vi "Delay in DDS.vi"() -> ()   [LabVIEW 2014]
uses:
  <vilib>/Platform/TimedLoop/XDataNode/timing_clust.ctl
  <vilib>/Platform/TimedLoop/XDataNode/nitl_modes.ctl
  <vilib>/Platform/TimedLoop/XDataNode/wakeup.ctl
  <vilib>/platform/TimedLoop/XDataNode/XDataNode.xnode
  <vilib>/Platform/TimedLoop/XDataNode/XDNodeRunTimeDep.lvlib
panel:
  out "x-y":u32
  out "millisecond timer value 2":u32
  out "millisecond timer value":u32
  out "Source vs PLC":cluster{"Value":dbl, "Value":dbl}(graph)
  out "PLC":dbl(graph)
  in  "PLC Scan Time":i64
  in  "DDS Update Rate":i64
  out "DDS":dbl(graph)
  out "Source":dbl(graph)
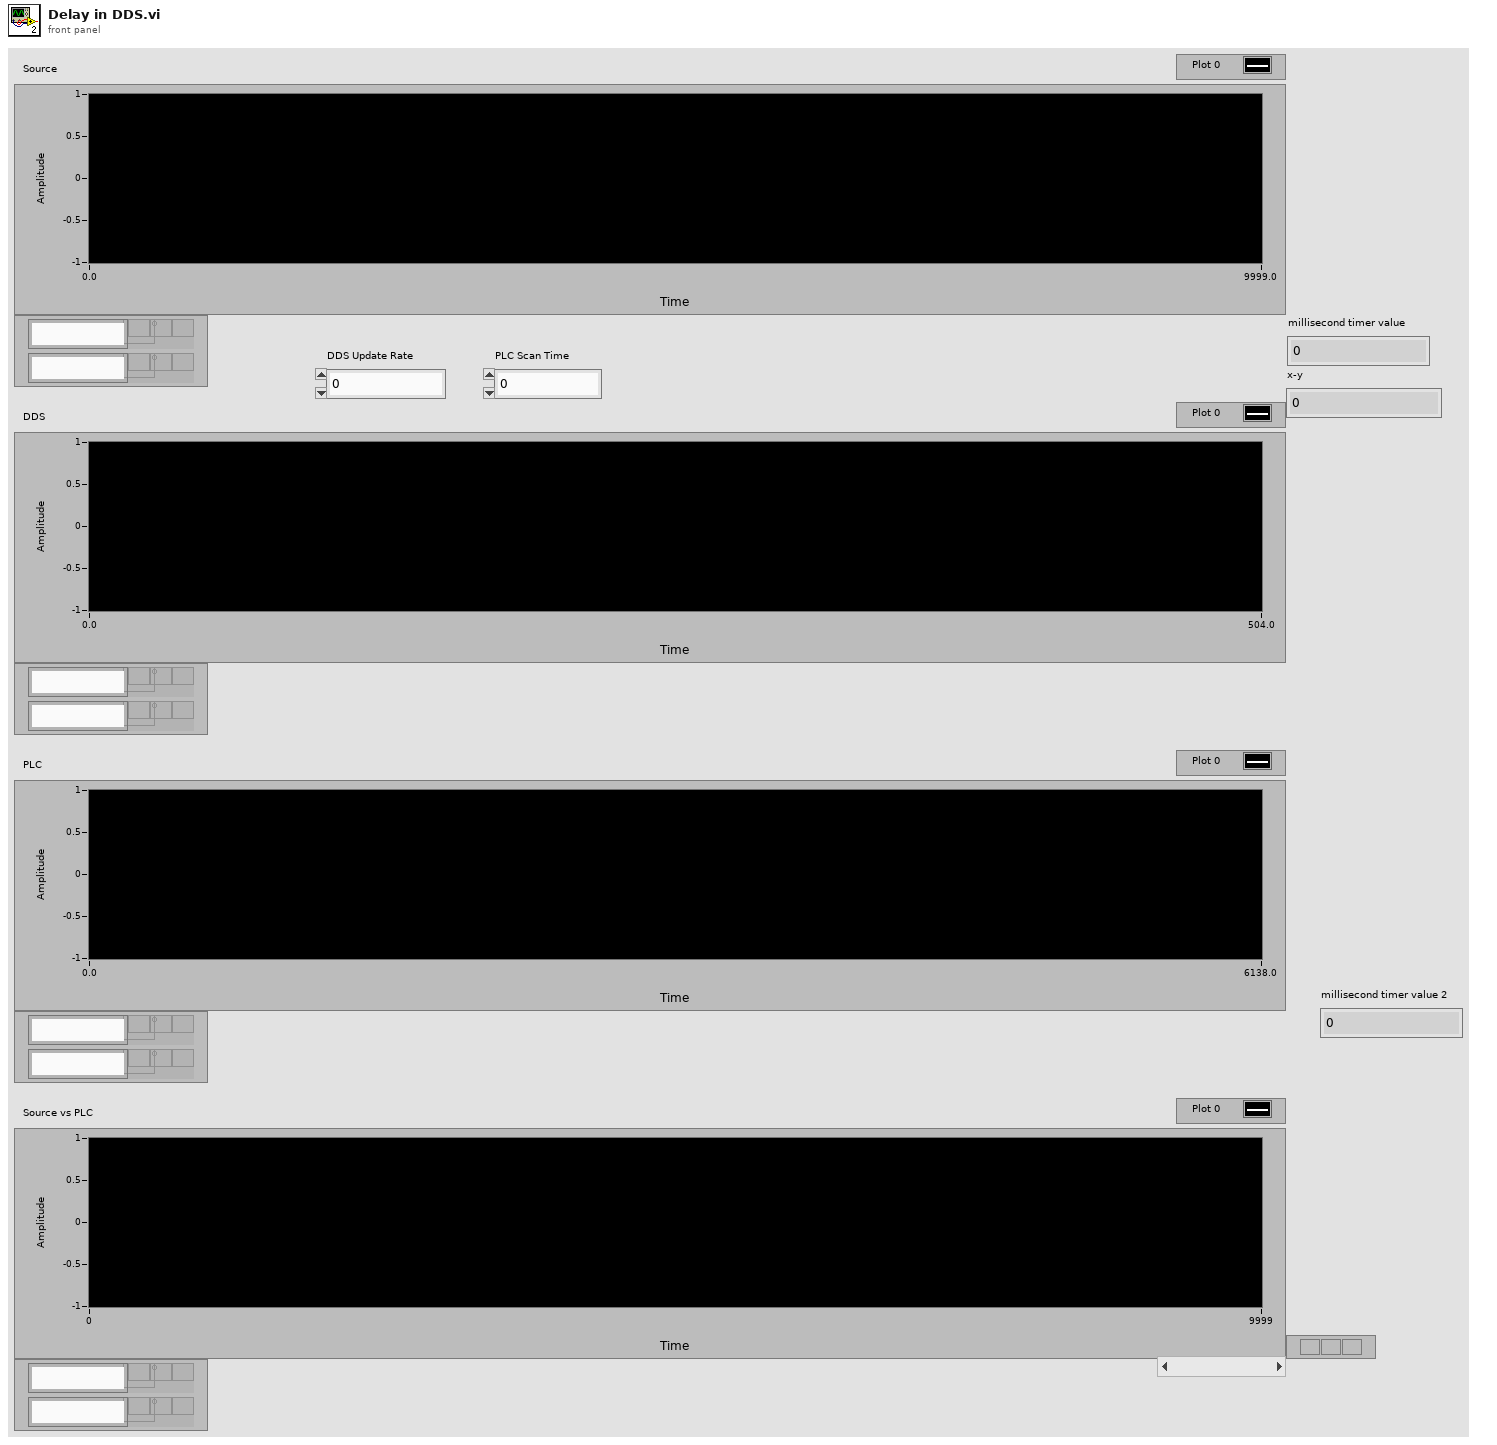
[diagram p1: front panel]
types:
  T1 = typedef "XDNodeRunTimeDep.lvlib/timing_clust.ctl" = cluster{"Expected End [f-1]":u64, "Actual End [f-1]":u64, "Finished Late? [f-1]":bool, "Expected End [i-1]":u64, "Actual End [i-1]":u64, "Finished Late? [i-1]":bool, "Expected Start [i]":u64, "Actual Start [i]":u64, "Expected Start [f]":u64, "Actual Start [f]":u64, "Source Name":string, "Structure Name":string, "Period":i64, "Deadline":i64, "Offset":i64, "Start":i64, "Priority":i32, "Timeout":i32, "Mode":T2, "Wakeup Reason":T3, "Error":errorcluster, "Source Type":string, "Secondary Source Type":string, "Global End Time":u64, "Global Start Time":u64, "Frame Duration":u64, "Iteration Duration":u64, "Assigned CPU":i32, "I/O Scan Engine Mode":u32}
  T2 = typedef "XDNodeRunTimeDep.lvlib/nitl_modes.ctl" = enum32{"No Change", "Process missed periods, maintain original phase", "Discard missed periods, maintain original phase", "Process missed periods, ignore original phase", "Discard missed periods, ignore original phase"}
  T3 = typedef "XDNodeRunTimeDep.lvlib/wakeup.ctl" = enum32{"Normal", "Aborted", "Asynchronous wakeup", "Timing source error", "Timed loop error", "Timeout"}
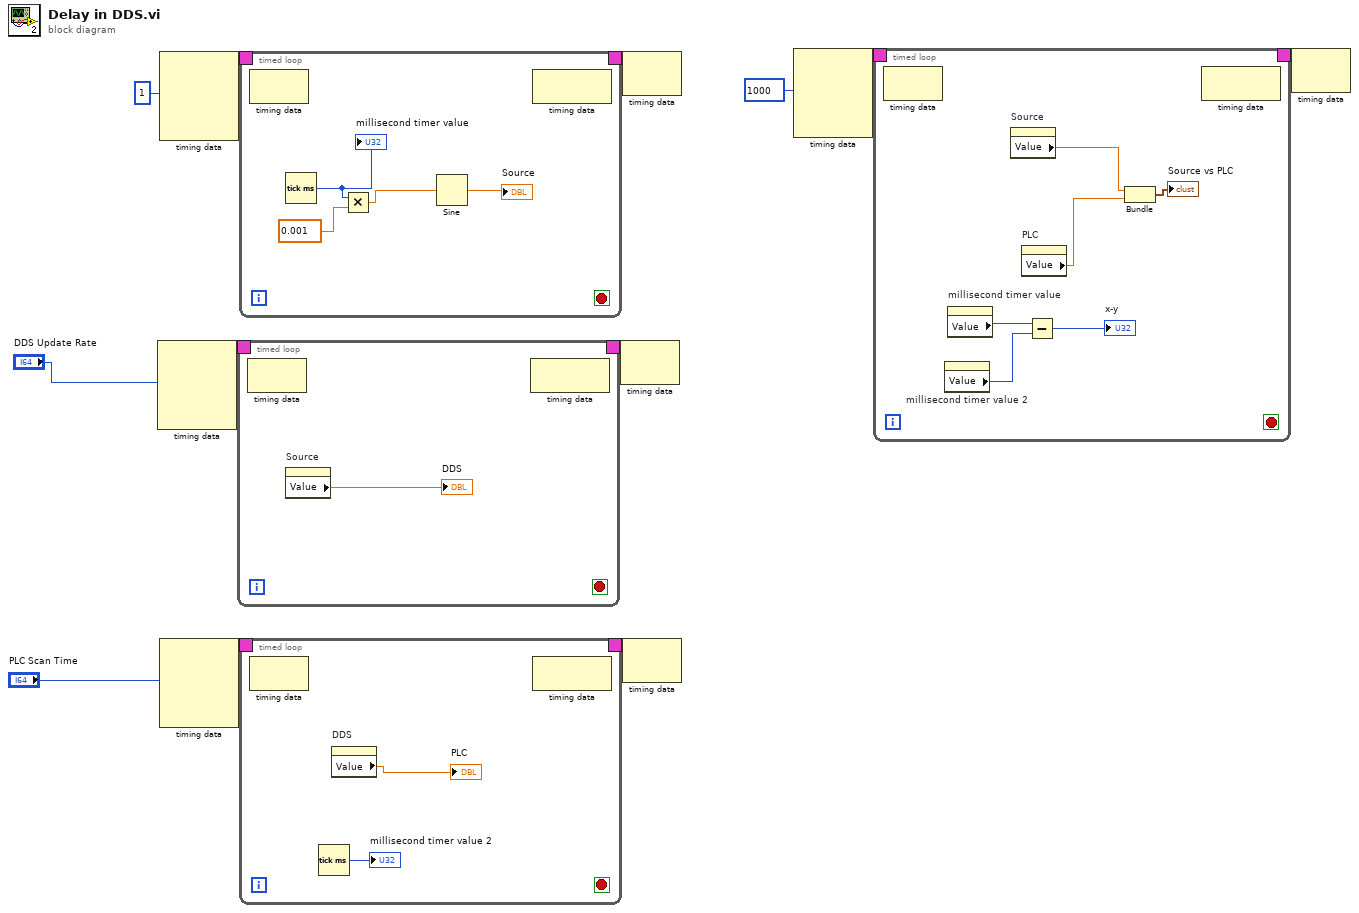
[diagram p0: block diagram]
diagram:
  n1 = node-c288("DDS Update Rate") -> (w10:T1)  [unwired: 3 in]
  n2 = node-c288(i64 1 ("Period")) -> (w12:T1)  [unwired: 3 in]
  n3 = node-c288("PLC Scan Time") -> (w8:T1)  [unwired: 3 in]
  n4 = timed-loop {
    timing: w10 -> [_]
    timing-out: [_] -> w9
    stop <- _ stop-if-true
    n5 = node-c288() -> ()  [unwired: 1 in, 1 out]
    n6 = property on="Source" class="WFChart (strict)"() -> ("Value"=→"DDS":dbl)  [unwired: 2 in, 2 out]
    n7 = node-c288() -> ()  [unwired: 1 in, 1 out]
  }
  n8 = timed-loop {
    timing: w12 -> [_]
    timing-out: [_] -> w11
    stop <- _ stop-if-true
    n9 = node-c288() -> ()  [unwired: 1 in, 1 out]
    n10 = Tick Count (ms)() -> (millisecond timer value=w18:u32)
    "millisecond timer value" <- w18
    n11 = Multiply(x=w18, y=0.001) -> (x*y=w17:dbl)
    n12 = Sine(x=w17) -> (sin(x)=→"Source":dbl)
    n13 = node-c288() -> ()  [unwired: 1 in, 1 out]
  }
  n14 = timed-loop {
    timing: w8 -> [_]
    timing-out: [_] -> w7
    stop <- _ stop-if-true
    n15 = node-c288() -> ()  [unwired: 1 in, 1 out]
    n16 = Tick Count (ms)() -> (millisecond timer value=→"millisecond timer value 2":u32)
    n17 = property on="DDS" class="WFChart (strict)"() -> ("Value"=→"PLC":dbl)  [unwired: 2 in, 2 out]
    n18 = node-c288() -> ()  [unwired: 1 in, 1 out]
  }
  n19 = node-c288(w9) -> ()  [unwired: 1 out]
  n20 = node-c288(w11) -> ()  [unwired: 1 out]
  n21 = node-c288(w7) -> ()  [unwired: 1 out]
  n22 = node-c288(i64 1000 ("Period")) -> (w3:T1)  [unwired: 3 in]
  n23 = timed-loop {
    timing: w3 -> [_]
    timing-out: [_] -> w2
    stop <- _ stop-if-true
    n24 = node-c288() -> ()  [unwired: 1 in, 1 out]
    n25 = property on="millisecond timer value 2" class="DigNum (strict)"() -> ("Value"=w27:u32)  [unwired: 2 in, 2 out]
    n26 = property on="millisecond timer value" class="DigNum (strict)"() -> ("Value"=w28:u32)  [unwired: 2 in, 2 out]
    n27 = property on="Source" class="WFChart (strict)"() -> ("Value"=w31:dbl)  [unwired: 2 in, 2 out]
    n28 = property on="PLC" class="WFChart (strict)"() -> ("Value"=w30:dbl)  [unwired: 2 in, 2 out]
    n29 = Subtract(x=w28, y=w27) -> (x-y=→"x-y":u32)
    n30 = Bundle("Value"=w31, "Value"=w30) -> (→"Source vs PLC":cluster{"Value":dbl, "Value":dbl})  [unwired: 1 in]
    n31 = node-c288() -> ()  [unwired: 1 in, 1 out]
  }
  n32 = node-c288(w2) -> ()  [unwired: 1 out]
